vi "SetAmpl.vi"(4 "Enable Attenuator Bypass":bool, 5 "Attenuation Level (dB)":dbl=115.0, 6 "Attenuator Auto Mode":bool=TRUE, 7 "Power Reference (dBm)":dbl, 8 "error in (no error)":errorcluster, 9 "Power Offset (dB)":dbl, 10 "Power (dBm)":dbl=-130.0, 11 "SigGen_MXG in":refnum<class "SigGen_MXG.lvclass">) -> (0 "error out":errorcluster, 3 "SigGen_MXG out":refnum<class "SigGen_MXG.lvclass">)   [LabVIEW 2014, in "SigGen_MXG.lvclass"]
uses:
  SigGen_MXG.lvclass
  SigGen_MXG.lvclass/SigGen_MXG.ctl
  <instrlib>/Agilent PSG MXG Series/Agilent PSG MXG Series.lvlib
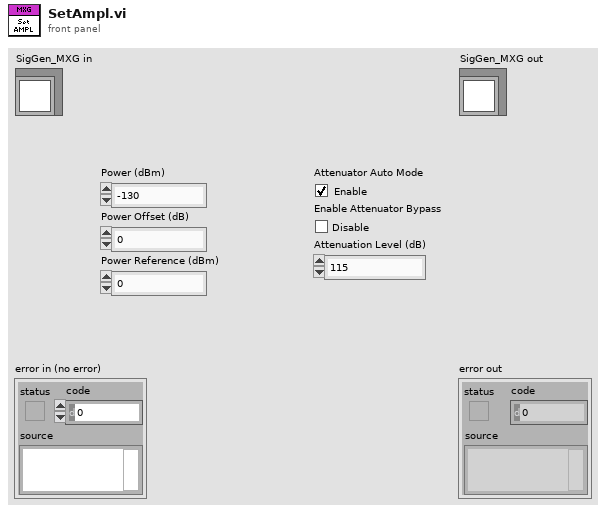
[diagram p1: front panel]
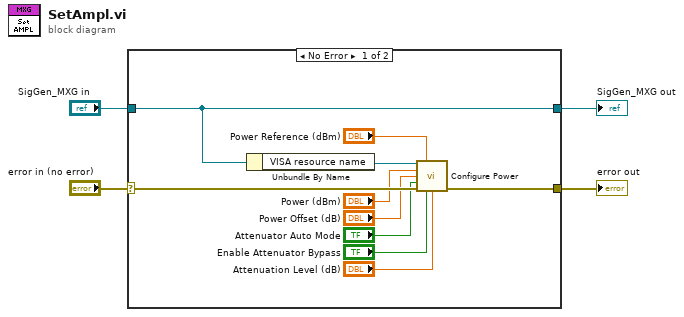
[diagram p0: block diagram]
diagram:
  n1 = case shown="No Error" "error in (no error)" {
    selector: "error in (no error)" -> [w14 w16]
    tunnel: [w13 w16] -> w3
    tunnel: [w12 w15] -> w1
    tunnel: "SigGen_MXG in" -> [w12 w15]
    frame No Error {
      n2 = Unbundle By Name(w12) -> ("VISA resource name"=w11:refnum<visa-resource-name>)
      n3 = call <instrlib>:"Configure Power.vi"("VISA resource name"=w11, "Power Reference (0 dBm)"="Power Reference (dBm)", "Power (-130 dBm)"="Power (dBm)", "Power Offset (0 dB)"="Power Offset (dB)", "Attenuator Auto Mode (T:Enable)"="Attenuator Auto Mode", "error in (no error)"=w14, "Enable Attenuator Bypass (F:Disable)"="Enable Attenuator Bypass", "Attenuation Level (115 dB)"="Attenuation Level (dB)") -> ("error out"=w13:errorcluster)  [unwired: 2 in, 5 out]
    }
    frame Error {
    }
  }
  "error out" <- w3
  "SigGen_MXG out" <- w1
